vi "-1开平方.vi"() -> ()   [LabVIEW 2020]
panel:
  out "复数":cdb=-1.0+0.0i
  out "开平方后的结果":dbl format="%#_13g"
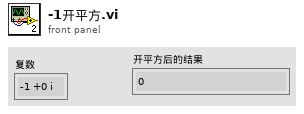
[diagram p1: front panel]
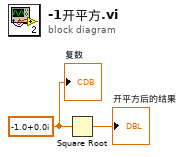
[diagram p0: block diagram]
diagram:
  w2 = cdb -1.0+0.0i
  n1 = Square Root(x=w2) -> (sqrt(x)=→"开平方后的结果":cdb)
  "复数" <- w2
